vi "RT Main v0.9.vi"() -> ()   [LabVIEW 2017]
doc: "Changelog:\n\nv0.9:\n- Autocycle"
uses:
  Controls/Auto Delays.ctl
  support/Controls/All Inputs.ctl
  support/Controls/Index Details.ctl
  support/Controls/Auto Stats.ctl
  Controls/Auto Times.ctl
  Global Variables/RT GV.vi
  support/Message Queue/Enqueue Message (Single).vi
  Global Variables/FPGA GV.vi
  <vilib>/Utility/error.llb/Error Cluster From Error Code.vi
  <vilib>/rvi/errors/niLvFpgaAdjustHostInterfaceError.vi
  Global Variables/Network Globals.vi
  <vilib>/FPGAPlugInAG/Dynamic/niLvFpga_Close_Dynamic.vi
  <vilib>/rvi/interface/nirviReadWriteControl/nirviReadWriteControl.xnode
  Controls/FPGA Ref.ctl
  <vilib>/rvi/interface/nirviCloseFPGA/nirviCloseFPGA.xnode
  support/Message Queue/Message Queue.lvlib
  NiFpgaLv.dll
  <vilib>/rvi/interface/Simulation/niFpgaSimulationCallBeginRW.vi
panel:
  in  "Auto Para":T1={"Agitator Delays"=[700, 250], "TF Delays"=[700, 800, 2], "Insertion Delays"=[100, 500], "Cutting Delays"=[300, 300, 100], "PF Delays"=[250, 30000], "Measur. Delays"=[500.0, 188.9, 1.0], "Reject Delays"=[500], "BF Delays"=[1000, 1000]}
  in  "Counts in":cluster{"OutputCount":u32, "RejectCount":u32}
  in  "Stop Button 4":bool
  out "error out":errorcluster
  out "Wrong Message":string
  in  "Stop Button":bool
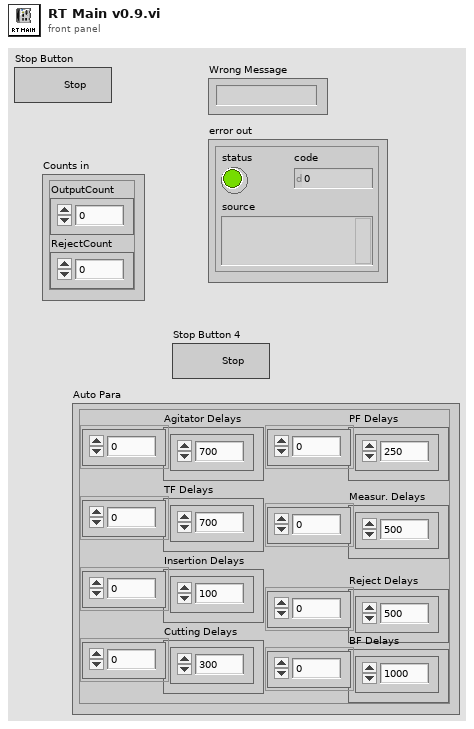
[diagram p1: front panel]
types:
  T1 = typedef "Auto Delays.ctl" = cluster{"Agitator Delays":u32[], "TF Delays":u32[], "Insertion Delays":u32[], "Cutting Delays":u32[], "PF Delays":u32[], "Measur. Delays":dbl[], "Reject Delays":u32[], "BF Delays":u32[]}
  T2 = typedef "FPGA Ref.ctl" = refnum<k20>
  T3 = cluster{"TL_Red":bool, "TL_Orange":bool, "TL_Green":bool, "TL_Buzzer":bool, "SOL_Index_Rotary_CW":bool, "SOL_Index_CNVR_Rotary_CCW":bool, "SOL_Index_CNVR_Stopper_Rear":bool, "SOL_Index_CNVR_Output _Separator _Rear":bool, "Bowl  Feeder_ ON":bool, "Pump_CNVR_Motor _ON":bool, "SOL_Gating_CYL_Rear":bool, "SOL_Tube_Feed_Agitatator":bool, "SOL_Tube_Feed_Gating_CYL":bool, "SOL_Insertion _CYL":bool, "SOL_Insertion_Clamp_CYL":bool, "SOL_Cutting_CYL":bool, "SOL_Cutting_Clamp_CYL":bool, "SOL_Insertion_Air_Nozzle":bool, "SOL_Measurement_CYL":bool, "SOL_Measure_Clamp_CYL":bool, "SOL_Rejection CYL_1":bool, "SOL_Rejection CYL_2":bool, "SOL_Rejection CYL_3":bool, "SOL_Rejection CYL_4":bool, "DO1.24":bool, "DO1.25":bool, "DO1.26":bool, "DO1.27":bool, "DO1.28":bool, "DO1.29":bool, "DO1.30":bool, "DO1.31":bool}
  T4 = typedef "All Inputs.ctl" = cluster{"DI 1":cluster{"Machine_ON":bool, "E_stop ":bool, "SW_Pressure":bool, "SW_Start ":bool, "SW_Reset":bool, "SW_Stop":bool, "SW_Door":bool, "RS_Index_Rotary_CW":bool, "RS_Index_Rotary_CCW":bool, "RS_Index_Stopper _Rear":bool, "RS_Index_Output_Separator_Rear":bool, "PES_Index_Pallet_Sensor":bool, "PES_Index_Output_Part Sensor":bool, "ICS_BF_Low_Level_1":bool, "ICS_BF_Low_Level_2":bool, "ICS_BF_Pump_CNVR_Full_1":bool, "ICS_BF_Pump_CNVR_Full_2":bool, "ICS_BF_Pump_CNVR_Full_3":bool, "ICS_BF_Pump_CNVR_Full_4":bool, "PES_PC_Pump Presence_1":bool, "PES_PC_Pump Presence_2":bool, "PES_PC_Pump Presence_3":bool, "PES_PC_Pump Presence_4":bool, "RS_PC_Gating_Front":bool, "PES_Pump_Interference":bool, "PES_TF_Low_Level":bool, "PES_Tube Presence_1":bool, "PES_Tube Presence_2":bool, "PES_Tube Presence_3":bool, "PES_Tube Presence_4":bool, "DI1.30":bool, "DI1.31":bool}, "DI 2":cluster{"RS_Agitatator_1_Rear ":bool, "RS_Agitatator_2_Rear ":bool, "RS_TF_Gating CYL_Rear":bool, "RS_Insertion_1_Rear":bool, "RS_Insertion_1_Front":bool, "RS_Insertion _2_Rear":bool, "RS_Insertion _2_Front":bool, "RS_Insertion _3_Rear":bool, "RS_Insertion _3_Front":bool, "RS_Insertion _4_Rear":bool, "RS_Insertion _4_Front":bool, "RS_Insertion_Clamp_Rear":bool, "RS_Cutting_Rear":bool, "RS_Cutting_Clamp _Rear":bool, "RS_Measurement_1_Rear":bool, "RS_Measurement_2_Rear":bool, "RS_Measurement_3_Rear":bool, "RS_Measurement_4_Rear":bool, "RS_Measure_Clamp_Rear":bool, "RS_Rejection_1_Rear":bool, "RS_Rejection_2_Rear":bool, "RS_Rejection_3_Rear":bool, "RS_Rejection_4_Rear":bool, "DI2.23":bool, "DI2.24":bool, "DI2.25":bool, "DI2.26":bool, "DI2.27":bool, "DI2.28":bool, "DI2.29":bool, "DI2.30":bool, "DI2.31":bool}, "IAS 1":dbl, "IAS 2":dbl, "IAS 3":dbl, "IAS 4":dbl, "DO 1":cluster{"TL_Red":bool, "TL_Orange":bool, "TL_Green":bool, "TL_Buzzer":bool, "SOL_Index_Rotary_CW":bool, "SOL_Index_CNVR_Rotary_CCW":bool, "SOL_Index_CNVR_Stopper_Rear":bool, "SOL_Index_CNVR_Output _Separator _Rear":bool, "Bowl  Feeder_ ON 1":bool, "Pump_CNVR_Motor _ON":bool, "SOL_PC_Gating_CYL_Rear":bool, "SOL_Tube_Feed_Agitatator":bool, "SOL_Tube_Feed_Gating_CYL":bool, "SOL_Insertion _CYL":bool, "SOL_Insertion_Clamp_CYL":bool, "SOL_Cutting_CYL":bool, "SOL_Cutting_Clamp_CYL":bool, "SOL_Insertion_Air_Nozzle":bool, "SOL_Measurement_CYL":bool, "DO1.19":bool, "SOL_Rejection CYL_1":bool, "SOL_Rejection CYL_2":bool, "SOL_Rejection CYL_3":bool, "SOL_Rejection CYL_4":bool, "Bowl  Feeder_ ON 2":bool, "SOL_BF_BlowerON":bool, "SOL_BF1_Track1":bool, "SOL_BF1_Track2":bool, "SOL_BF2_Track1":bool, "SOL_BF2_Track2":bool, "DO1.30":bool, "DO1.31":bool}}
  T5 = typedef "Index Details.ctl" = cluster{"Time (ms)":u32, "Waveform Graph":i16[]}
  T6 = cluster{T1, "Reject Pallets":cluster{"Reject 1":bool, "Reject 2":bool, "Reject 3":bool, "Reject 4":bool}}
  T7 = typedef "Auto Stats.ctl" = cluster{"Time":timestamp, "OEE":cluster{"AVL":dbl, "PRF":dbl, "QUA":dbl, "OEE":dbl}, "Auto Times":T8, "Counts out":cluster{"OutputCount":u32, "RejectCount":u32}, "Measurements":cluster{"1":dbl, "2":dbl, "3":dbl, "4":dbl}, "Outputs":cluster{"OutputCount":u32, "Numeric Control":u32}}
  T8 = typedef "Auto Times.ctl" = cluster{"Index Time":u32, "TF Time":u32, "Insertion Time":u32, "Cutting Time":u32, "PF Time":u32, "Meas. Time":u32, "Reject Time":u32}
  T9 = cluster{string, dbl, "Counts in":cluster{"OutputCount":u32, "RejectCount":u32}, "Auto Para":T1}
  T10 = cluster{"TL_Red":bool, "TL_Orange":bool, "TL_Green":bool, "TL_Buzzer":bool, "SOL_Index_Rotary_CW":bool, "SOL_Index_CNVR_Rotary_CCW":bool, "SOL_Index_CNVR_Stopper_Rear":bool, "SOL_Index_CNVR_Output _Separator _Rear":bool, "Bowl Feeder_ ON1":bool, "Pump_CNVR_Motor _ON":bool, "SOL_PC_Gating_CYL_Rear":bool, "SOL_Tube_Feed_Agitatator":bool, "SOL_Tube_Feed_Gating_CYL":bool, "SOL_Insertion _CYL":bool, "SOL_Insertion_Clamp_CYL":bool, "SOL_Cutting_CYL":bool, "SOL_Cutting_Clamp_CYL":bool, "SOL_Insertion_Air_Nozzle":bool, "SOL_Measurement_CYL":bool, "DO1.19":bool, "SOL_Rejection CYL_1":bool, "SOL_Rejection CYL_2":bool, "SOL_Rejection CYL_3":bool, "SOL_Rejection CYL_4":bool, "Bowl Feeder_ON2":bool, "SOL_BF_BlowerON":bool, "SOL_BF1_Track1":bool, "SOL_BF1_Track2":bool, "SOL_BF2_Track1":bool, "SOL_BF2_Track2":bool, "DO1.30":bool, "DO1.31":bool}
  T11 = cluster{"Machine_ON":bool, "E_stop ":bool, "SW_Pressure":bool, "SW_Start ":bool, "SW_Reset":bool, "SW_Stop":bool, "SW_Door":bool, "RS_Index_Rotary_CW":bool, "RS_Index_Rotary_CCW":bool, "RS_Index_Stopper _Rear":bool, "RS_Index_Output_Separator_Rear":bool, "PES_Index_Pallet_Sensor":bool, "PES_Index_Output_Part Sensor":bool, "ICS_BF_Low_Level_1":bool, "ICS_BF_Low_Level_2":bool, "ICS_BF_Pump_CNVR_Full_1":bool, "ICS_BF_Pump_CNVR_Full_2":bool, "ICS_BF_Pump_CNVR_Full_3":bool, "ICS_BF_Pump_CNVR_Full_4":bool, "PES_PC_Pump Presence_1":bool, "PES_PC_Pump Presence_2":bool, "PES_PC_Pump Presence_3":bool, "PES_PC_Pump Presence_4":bool, "RS_PC_Gating_Front":bool, "PES_Pump_Interference":bool, "PES_TF_Low_Level":bool, "PES_Tube Presence_1":bool, "PES_Tube Presence_2":bool, "PES_Tube Presence_3":bool, "PES_Tube Presence_4":bool, "DI1.30":bool, "DI1.31":bool}
  T12 = cluster{"RS_Agitatator_1_Rear ":bool, "RS_Agitatator_2_Rear ":bool, "RS_TF_Gating CYL_Rear":bool, "RS_Insertion_1_Rear":bool, "RS_Insertion_1_Front":bool, "RS_Insertion _2_Rear":bool, "RS_Insertion _2_Front":bool, "RS_Insertion _3_Rear":bool, "RS_Insertion _3_Front":bool, "RS_Insertion _4_Rear":bool, "RS_Insertion _4_Front":bool, "RS_Insertion_Clamp_Rear":bool, "RS_Cutting_Rear":bool, "RS_Cutting_Clamp _Rear":bool, "RS_Measurement_1_Rear":bool, "RS_Measurement_2_Rear":bool, "RS_Measurement_3_Rear":bool, "RS_Measurement_4_Rear":bool, "DI2.18":bool, "RS_Rejection_1_Rear":bool, "RS_Rejection_2_Rear":bool, "RS_Rejection_3_Rear":bool, "RS_Rejection_4_Rear":bool, "DI2.23":bool, "DI2.24":bool, "DI2.25":bool, "DI2.26":bool, "DI2.27":bool, "DI2.28":bool, "DI2.29":bool, "DI2.30":bool, "DI2.31":bool}
  T13 = cluster{"Array":string[][], "Machine Status":string}
  T14 = cluster{"Measurements":cluster{"1":dbl, "2":dbl, "3":dbl, "4":dbl}, "Reject Pallets":cluster{"Reject 1":bool, "Reject 2":bool, "Reject 3":bool, "Reject 4":bool}}
  T15 = cluster{"Auto Times":T8, "Results":cluster{"Measurements":cluster{"1":dbl, "2":dbl, "3":dbl, "4":dbl}, "Reject Pallets":cluster{"Reject 1":bool, "Reject 2":bool, "Reject 3":bool, "Reject 4":bool}}, "OutputCount":u32, "error out":errorcluster}
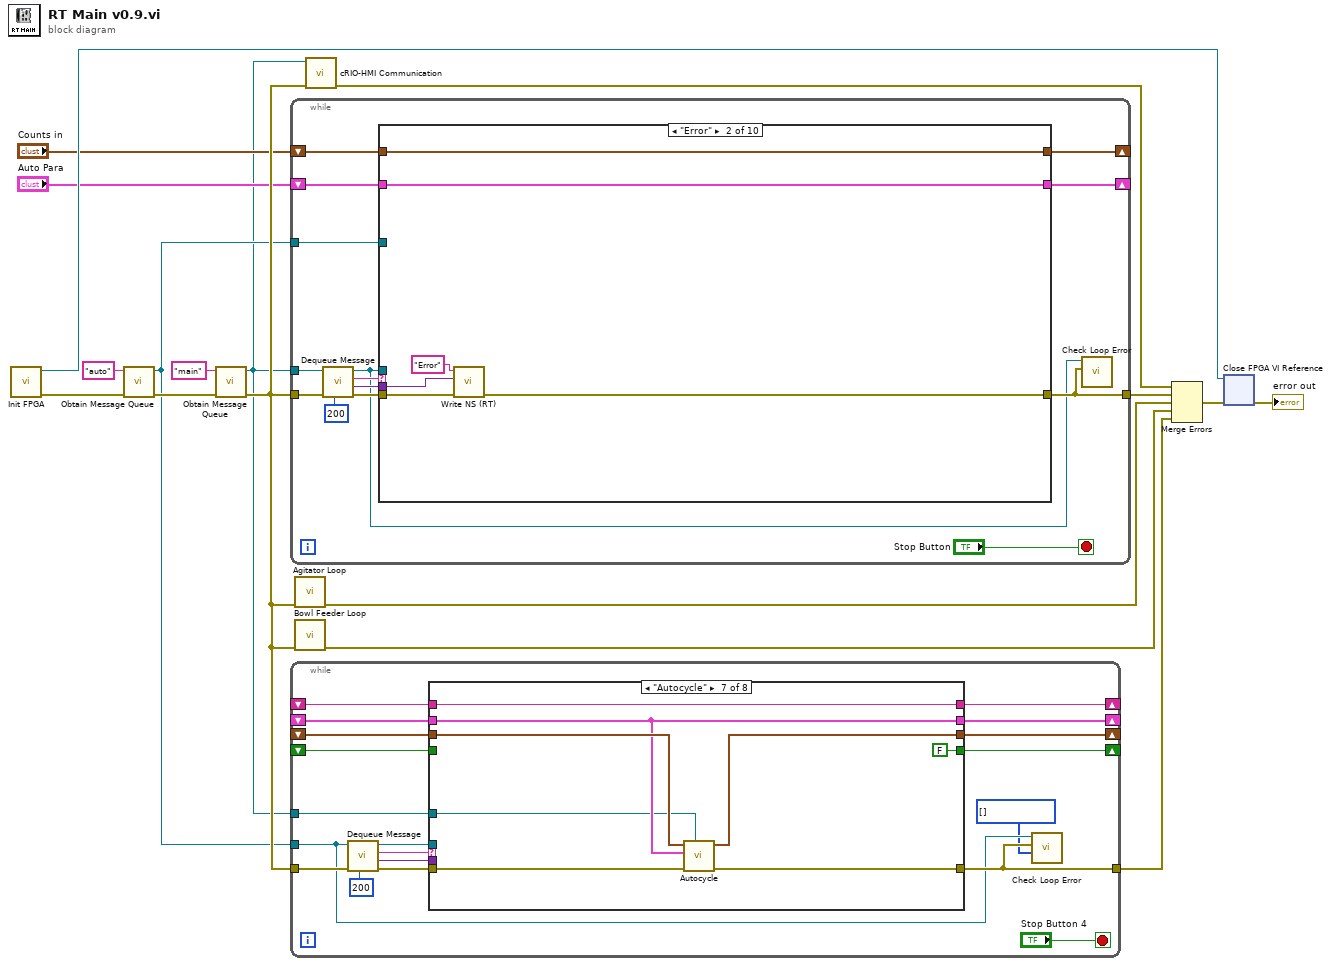
[diagram p0: block diagram]
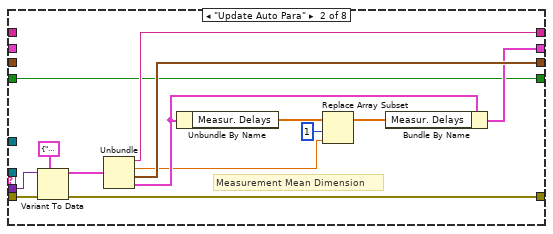
[diagram p3: hidden frame]
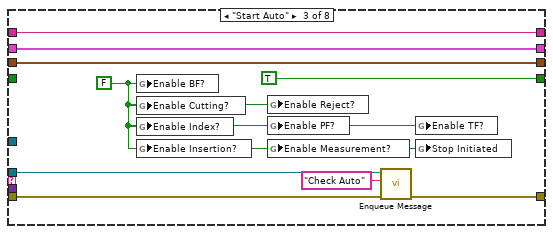
[diagram p4: hidden frame]
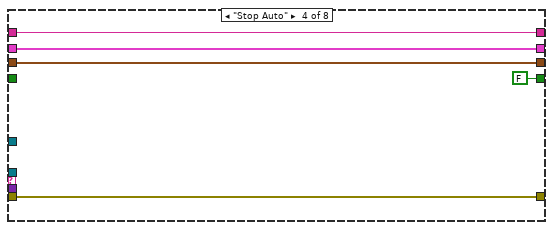
[diagram p5: hidden frame]
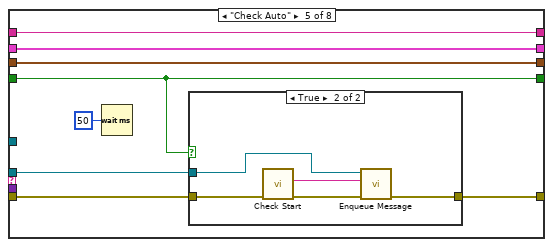
[diagram p6: hidden frame]
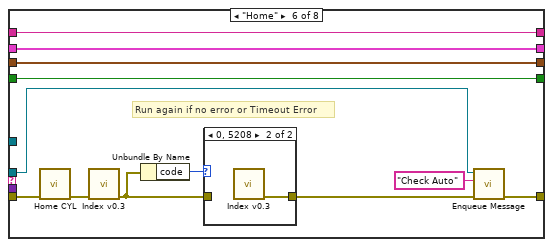
[diagram p8: hidden frame]
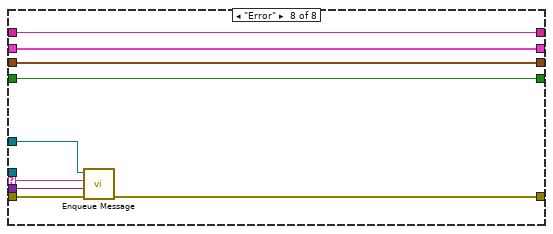
[diagram p10: hidden frame]
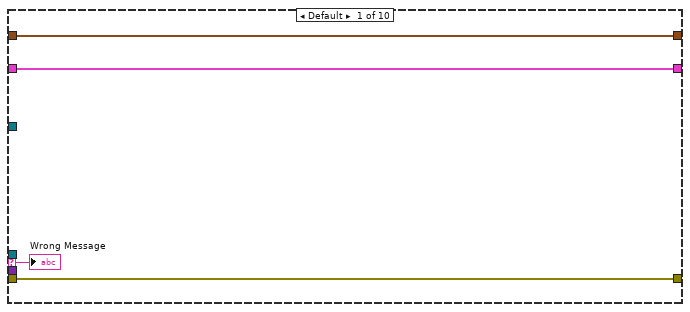
[diagram p11: hidden frame]
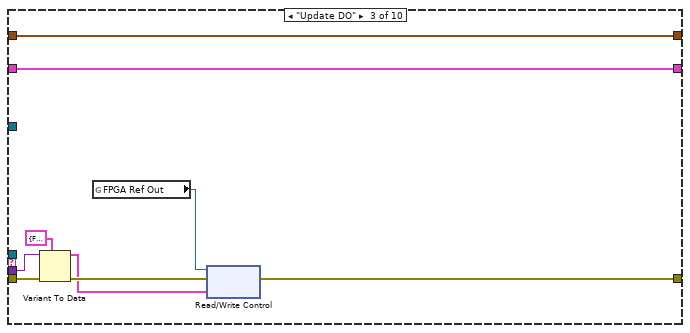
[diagram p12: hidden frame]
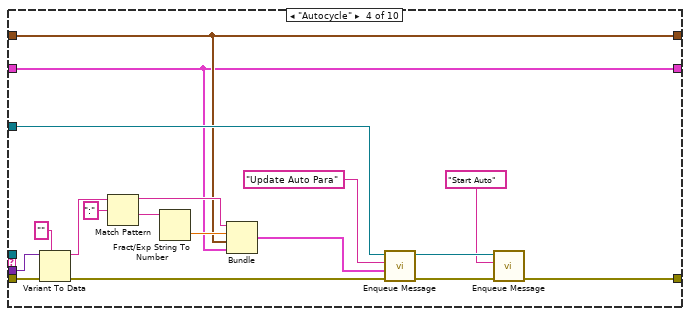
[diagram p13: hidden frame]
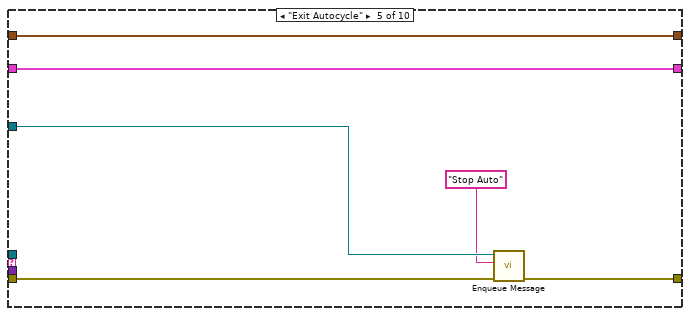
[diagram p14: hidden frame]
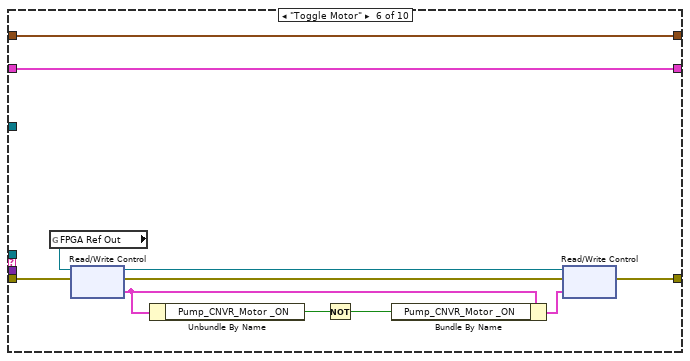
[diagram p15: hidden frame]
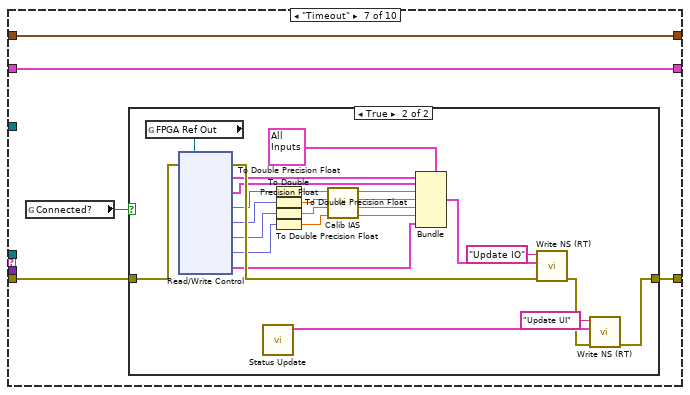
[diagram p16: hidden frame]
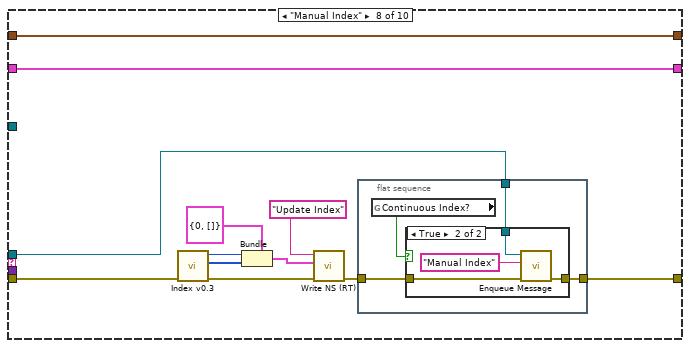
[diagram p18: hidden frame]
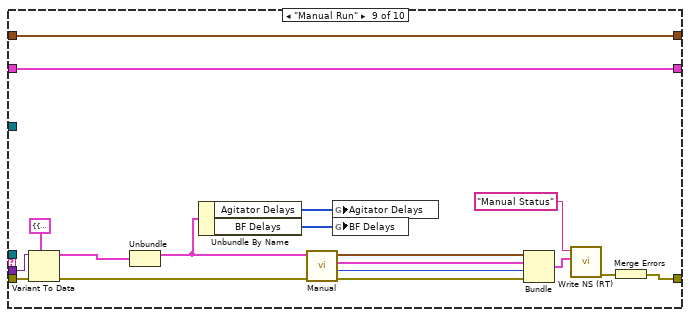
[diagram p20: hidden frame]
diagram:
  n1 = call "Init FPGA.vi"() -> ("error out"=w6:errorcluster, "FPGA Ref Out"=w11:T2)  [unwired: 10 in]
  n2 = call "Obtain Message Queue.vi"("error in (no error)"=w6, "name"="auto") -> ("error out"=w5:errorcluster, "Message Queue"=w2:refnum<queue>)  [unwired: 8 in]
  n3 = call "Obtain Message Queue.vi"("error in (no error)"=w5, "name"="main") -> ("error out"=w10:errorcluster, "Message Queue"=w1:refnum<queue>)  [unwired: 8 in]
  n4 = while {
    tunnel: w10 -> [w30]
    tunnel: w1 -> [w29]
    tunnel: [w25] -> w17
    tunnel: w2 -> [w22]
    shift-right: [w19] -> _
    shift-left: "Auto Para" -> [w20]
    shift-right: [w18] -> _
    shift-left: "Counts in" -> [w21]
    stop <- "Stop Button" stop-if-true
    n5 = call "Dequeue Message.vi"("timeout"=200, "error in (no error)"=w30, "Message Queue"=w29) -> ("error out"=w28:errorcluster, "Message Data"=w26:variant, "Message"=w27:string, "dup Message Queue"=w24:refnum<queue>)  [unwired: 5 in]
    n6 = case shown="\"Error\"" w27 {
      selector: w27 -> [w35 _ _ _ _ _ _ _ _ _]
      tunnel: w28 -> [w34 w39 w50 w68 w74 w84 w89 w128 w155 w165]
      tunnel: w24 -> [_ _ _ _ _ _ _ w120 _ _]
      tunnel: w26 -> [_ w37 w49 w67 _ _ _ _ w154 w164]
      tunnel: [w34 w38 w45 w53 w70 w82 w90 w121 w150 w161] -> w25
      tunnel: w22 -> [_ _ _ w60 w73 _ _ _ _ _]
      tunnel: w21 -> [w33 w41 w43 w57 w72 w76 w87 w117 w141 w160]
      tunnel: w20 -> [w32 w40 w42 w56 w71 w75 w86 w118 w140 w159]
      tunnel: [w32 w40 w42 w56 w71 w75 w86 w118 w140 w159] -> w19
      tunnel: [w33 w41 w43 w57 w72 w76 w87 w117 w141 w160] -> w18
      frame Default {
        "Wrong Message" <- w35
      }
      frame "Error" {
        n7 = call "Write NS (RT).vi"("error in (no error)"=w39, "Message Data"=w37, "Message"="Error") -> ("error out"=w38:errorcluster)  [unwired: 8 in]
      }
      frame "Update DO" {
        n8 = Variant To Data(error in=w50, type=T3 {"TL_Red"=FALSE, "TL_Orange"=FALSE, "TL_Green"=FALSE, "TL_Buzzer"=FALSE, "SOL_Index_Rotary_CW"=FALSE, "SOL_Index_CNVR_Rotary_CCW"=FALSE, "SOL_Index_CNVR_Stopper_Rear"=FALSE, "SOL_Index_CNVR_Output _Separator _Rear"=FALSE, "Bowl  Feeder_ ON"=FALSE, "Pump_CNVR_Motor _ON"=FALSE, "SOL_Gating_CYL_Rear"=FALSE, "SOL_Tube_Feed_Agitatator"=FALSE, "SOL_Tube_Feed_Gating_CYL"=FALSE, "SOL_Insertion _CYL"=FALSE, "SOL_Insertion_Clamp_CYL"=FALSE, "SOL_Cutting_CYL"=FALSE, "SOL_Cutting_Clamp_CYL"=FALSE, "SOL_Insertion_Air_Nozzle"=FALSE, "SOL_Measurement_CYL"=FALSE, "SOL_Measure_Clamp_CYL"=FALSE, "SOL_Rejection CYL_1"=FALSE, "SOL_Rejection CYL_2"=FALSE, "SOL_Rejection CYL_3"=FALSE, "SOL_Rejection CYL_4"=FALSE, "DO1.24"=FALSE, "DO1.25"=FALSE, "DO1.26"=FALSE, "DO1.27"=FALSE, "DO1.28"=FALSE, "DO1.29"=FALSE, "DO1.30"=FALSE, "DO1.31"=FALSE} ("DO 1"), Variant=w49) -> (data=w44:T3, error out=w46:errorcluster)
        n9 = global read "FPGA GV.vi" "FPGA Ref Out"() -> (w47:T2)
        n10 = xnode "Read/Write Control"("FPGA VI Reference In"=w47, "error in"=w46, "DO 1"=w44) -> ("error out"=w45:errorcluster)  [unwired: 1 out]
      }
      frame "Autocycle" {
        n11 = Variant To Data(error in=w68, type="", Variant=w67) -> (data=w63:string, error out=w61:errorcluster)
        n12 = Match Pattern(string=w63, regular expression=":") -> (before substring=w59:string, after substring=w64:string)  [unwired: 1 in, 2 out]
        n13 = Fract/Exp String To Number(string=w64) -> (number=w58:dbl)  [unwired: 3 in, 1 out]
        n14 = Bundle(w59, w58, "Counts in"=w57, "Auto Para"=w56) -> (w55:T9)  [unwired: 1 in]
        n15 = call-poly "Enqueue Message.vi"("error in (no error)"=w61, "Message Data"=w55, "Message"="Update Auto Para", "Message Queue"=w60) -> ("error out"=w54:errorcluster, "dup Message Queue"=w52:refnum<queue>)  [unwired: 6 in]
        n16 = call-poly "Enqueue Message.vi"("error in (no error)"=w54, "Message"="Start Auto", "Message Queue"=w52) -> ("error out"=w53:errorcluster)  [unwired: 7 in, 1 out]
      }
      frame "Exit Autocycle" {
        n17 = call-poly "Enqueue Message.vi"("error in (no error)"=w74, "Message"="Stop Auto", "Message Queue"=w73) -> ("error out"=w70:errorcluster)  [unwired: 7 in, 1 out]
      }
      frame "Toggle Motor" {
        n18 = global read "FPGA GV.vi" "FPGA Ref Out"() -> (w85:T2)
        n19 = xnode "Read/Write Control"("FPGA VI Reference In"=w85, "error in"=w84) -> ("FPGA VI Reference Out"=w81:T2, "error out"=w83:errorcluster, "DO 1"=w79:T10)
        n20 = Unbundle By Name(w79) -> ("Pump_CNVR_Motor _ON"=w80:bool)
        n21 = Not(x=w80) -> (.not. x?=w77:bool)
        n22 = Bundle By Name(cluster=w79, "Pump_CNVR_Motor _ON"=w77) -> (w78:T10)
        n23 = xnode "Read/Write Control"("FPGA VI Reference In"=w81, "error in"=w83, "DO 1"=w78) -> ("error out"=w82:errorcluster)  [unwired: 1 out]
      }
      frame "Timeout" {
        n24 = global read "Network Globals.vi" "Connected?"() -> (w88:bool)
        n25 = case shown="True" w88 {
          tunnel: [w91 w93] -> w90
          tunnel: w89 -> [w91 w115]
          frame False {
          }
          frame True {
            n26 = global read "FPGA GV.vi" "FPGA Ref Out"() -> (w92:T2)
            n27 = xnode "Read/Write Control"("FPGA VI Reference In"=w92, "error in"=w115) -> ("error out"=w114:errorcluster, "DI 1"=w113:T11, "DI 2"=w112:T12, "AI0"=w111:fxp<+/-,27,6>, "AI1"=w110:fxp<+/-,27,6>, "AI2"=w109:fxp<+/-,27,6>, "AI3"=w108:fxp<+/-,27,6>, "DO 1"=w105:T10)  [unwired: 1 out]
            n28 = call "Status Update.vi"() -> ("Status Cluster"=w95:T13)  [unwired: 11 in]
            n29 = To Double Precision Float(number=w111) -> (double precision float=w98:dbl)
            n30 = To Double Precision Float(number=w110) -> (double precision float=w100:dbl)
            n31 = To Double Precision Float(number=w109) -> (double precision float=w102:dbl)
            n32 = To Double Precision Float(number=w108) -> (double precision float=w104:dbl)
            n33 = call "Calib IAS.vi"("x 4"=w104, "x 3"=w102, "x 2"=w100, "x"=w98) -> ("y 4"=w103:dbl, "y 3"=w101:dbl, "y 2"=w99:dbl, "y 1"=w97:dbl)  [unwired: 4 in]
            n34 = Bundle(cluster=T4 {"DI 1"={"Machine_ON"=FALSE, "E_stop "=FALSE, "SW_Pressure"=FALSE, "SW_Start "=FALSE, "SW_Reset"=FALSE, "SW_Stop"=FALSE, "SW_Door"=FALSE, "RS_Index_Rotary_CW"=FALSE, "RS_Index_Rotary_CCW"=FALSE, "RS_Index_Stopper _Rear"=FALSE, "RS_Index_Output_Separator_Rear"=FALSE, "PES_Index_Pallet_Sensor"=FALSE, "PES_Index_Output_Part Sensor"=FALSE, "ICS_BF_Low_Level_1"=FALSE, "ICS_BF_Low_Level_2"=FALSE, "ICS_BF_Pump_CNVR_Full_1"=FALSE, "ICS_BF_Pump_CNVR_Full_2"=FALSE, "ICS_BF_Pump_CNVR_Full_3"=FALSE, "ICS_BF_Pump_CNVR_Full_4"=FALSE, "PES_PC_Pump Presence_1"=FALSE, "PES_PC_Pump Presence_2"=FALSE, "PES_PC_Pump Presence_3"=FALSE, "PES_PC_Pump Presence_4"=FALSE, "RS_PC_Gating_Front"=FALSE, "PES_Pump_Interference"=FALSE, "PES_TF_Low_Level"=FALSE, "PES_Tube Presence_1"=FALSE, "PES_Tube Presence_2"=FALSE, "PES_Tube Presence_3"=FALSE, "PES_Tube Presence_4"=FALSE, "DI1.30"=FALSE, "DI1.31"=FALSE}, "DI 2"={"RS_Agitatator_1_Rear "=FALSE, "RS_Agitatator_2_Rear "=FALSE, "RS_TF_Gating CYL_Rear"=FALSE, "RS_Insertion_1_Rear"=FALSE, "RS_Insertion_1_Front"=FALSE, "RS_Insertion _2_Rear"=FALSE, "RS_Insertion _2_Front"=FALSE, "RS_Insertion _3_Rear"=FALSE, "RS_Insertion _3_Front"=FALSE, "RS_Insertion _4_Rear"=FALSE, "RS_Insertion _4_Front"=FALSE, "RS_Insertion_Clamp_Rear"=FALSE, "RS_Cutting_Rear"=FALSE, "RS_Cutting_Clamp _Rear"=FALSE, "RS_Measurement_1_Rear"=FALSE, "RS_Measurement_2_Rear"=FALSE, "RS_Measurement_3_Rear"=FALSE, "RS_Measurement_4_Rear"=FALSE, "RS_Measure_Clamp_Rear"=FALSE, "RS_Rejection_1_Rear"=FALSE, "RS_Rejection_2_Rear"=FALSE, "RS_Rejection_3_Rear"=FALSE, "RS_Rejection_4_Rear"=FALSE, "DI2.23"=FALSE, "DI2.24"=FALSE, "DI2.25"=FALSE, "DI2.26"=FALSE, "DI2.27"=FALSE, "DI2.28"=FALSE, "DI2.29"=FALSE, "DI2.30"=FALSE, "DI2.31"=FALSE}, "IAS 1"=0.0, "IAS 2"=0.0, "IAS 3"=0.0, "IAS 4"=0.0, "DO 1"={"TL_Red"=FALSE, "TL_Orange"=FALSE, "TL_Green"=FALSE, "TL_Buzzer"=FALSE, "SOL_Index_Rotary_CW"=FALSE, "SOL_Index_CNVR_Rotary_CCW"=FALSE, "SOL_Index_CNVR_Stopper_Rear"=FALSE, "SOL_Index_CNVR_Output _Separator _Rear"=FALSE, "Bowl  Feeder_ ON 1"=FALSE, "Pump_CNVR_Motor _ON"=FALSE, "SOL_PC_Gating_CYL_Rear"=FALSE, "SOL_Tube_Feed_Agitatator"=FALSE, "SOL_Tube_Feed_Gating_CYL"=FALSE, "SOL_Insertion _CYL"=FALSE, "SOL_Insertion_Clamp_CYL"=FALSE, "SOL_Cutting_CYL"=FALSE, "SOL_Cutting_Clamp_CYL"=FALSE, "SOL_Insertion_Air_Nozzle"=FALSE, "SOL_Measurement_CYL"=FALSE, "DO1.19"=FALSE, "SOL_Rejection CYL_1"=FALSE, "SOL_Rejection CYL_2"=FALSE, "SOL_Rejection CYL_3"=FALSE, "SOL_Rejection CYL_4"=FALSE, "Bowl  Feeder_ ON 2"=FALSE, "SOL_BF_BlowerON"=FALSE, "SOL_BF1_Track1"=FALSE, "SOL_BF1_Track2"=FALSE, "SOL_BF2_Track1"=FALSE, "SOL_BF2_Track2"=FALSE, "DO1.30"=FALSE, "DO1.31"=FALSE}}, "DI 1"=w113, "DI 2"=w112, "IAS 1"=w97, "IAS 2"=w99, "IAS 3"=w101, "IAS 4"=w103, "DO 1"=w105) -> (w107:T4)
            n35 = call "Write NS (RT).vi"("error in (no error)"=w114, "Message Data"=w107, "Message"="Update IO") -> ("error out"=w94:errorcluster)  [unwired: 8 in]
            n36 = call "Write NS (RT).vi"("error in (no error)"=w94, "Message Data"=w95, "Message"="Update UI") -> ("error out"=w93:errorcluster)  [unwired: 8 in]
          }
        }
      }
      frame "Manual Index" {
        n37 = call "Index v0.3.vi"("error in (no error)"=w128) -> ("error out"=w126:errorcluster, "Waveform Graph"=w124:i16[], "Index Time"=w125:u32)  [unwired: 7 in, 1 out]
        n38 = Bundle(cluster=T5 {"Time (ms)"=0, "Waveform Graph"=[]}, "Time (ms)"=w125, "Waveform Graph"=w124) -> (w123:T5)
        n39 = call "Write NS (RT).vi"("error in (no error)"=w126, "Message Data"=w123, "Message"="Update Index") -> ("error out"=w122:errorcluster)  [unwired: 8 in]
        n40 = flat-sequence {
          tunnel: w122 -> [w132]
          tunnel: [w131] -> w121
          tunnel: w120 -> [w129]
          frame #0 {
            n41 = global read "RT GV.vi" "Continuous Index?"() -> (w130:bool)
            n42 = case shown="True" w130 {
              tunnel: w132 -> [w133 w137]
              tunnel: [w133 w136] -> w131
              tunnel: w129 -> [_ w134]
              frame False {
              }
              frame True {
                n43 = call-poly "Enqueue Message.vi"("error in (no error)"=w137, "Message"="Manual Index", "Message Queue"=w134) -> ("error out"=w136:errorcluster)  [unwired: 7 in, 1 out]
              }
            }
          }
        }
      }
      frame "Manual Run" {
        n44 = Variant To Data(error in=w155, type=T6 {{"Agitator Delays"=[1000], "TF Delays"=[1000], "Insertion Delays"=[1000], "Cutting Delays"=[1000], "PF Delays"=[1000], "Measur. Delays"=[1000.0], "Reject Delays"=[1000], "BF Delays"=[1000]}, "Reject Pallets"={"Reject 1"=FALSE, "Reject 2"=FALSE, "Reject 3"=FALSE, "Reject 4"=FALSE}}, Variant=w154) -> (data=w146:T6, error out=w153:errorcluster)
        n45 = Unbundle(w146) -> (w143:T1)  [unwired: 1 out]
        n46 = Unbundle By Name(w143) -> ("Agitator Delays"=w139:u32[], "BF Delays"=w138:u32[])
        n47 = call "Manual.vi"("error in"=w153, "Auto Delays"=w143) -> ("error out"=w145:errorcluster, "OutputCount"=w144:u32, "Results"=w142:T14, "Auto Times"=w149:T8)  [unwired: 6 in]
        n48 = global write "RT GV.vi" "Agitator Delays"(w139) -> ()
        n49 = global write "RT GV.vi" "BF Delays"(w138) -> ()
        n50 = Bundle("Auto Times"=w149, "Results"=w142, "OutputCount"=w144, "error out"=w145) -> (w148:T15)  [unwired: 1 in]
        n51 = call "Write NS (RT).vi"("Message Data"=w148, "Message"="Manual Status") -> ("error out"=w151:errorcluster)  [unwired: 9 in]
        n52 = Merge Errors(w151) -> (w150:errorcluster)
      }
      frame "Log Cycle" {
        n53 = Variant To Data(error in=w165, type=T7 {"Time"=timestamp(0 s since 1904-01-01), "OEE"={"AVL"=100.0, "PRF"=100.0, "QUA"=100.0, "OEE"=0.0}, "Auto Times"={"Index Time"=0, "TF Time"=0, "Insertion Time"=0, "Cutting Time"=0, "PF Time"=0, "Meas. Time"=0, "Reject Time"=0}, "Counts out"={"OutputCount"=0, "RejectCount"=0}, "Measurements"={"1"=0.0, "2"=0.0, "3"=0.0, "4"=0.0}, "Outputs"={"OutputCount"=0, "Numeric Control"=0}} ("Auto Stats"), Variant=w164) -> (data=w156:T7, error out=w157:errorcluster)
        n54 = call "Write NS (RT).vi"("error in (no error)"=w157, "Message Data"=w156, "Message"="Autocycle Log") -> ("error out"=w162:errorcluster)  [unwired: 8 in]
        n55 = Merge Errors(w162) -> (w161:errorcluster)
      }
    }
    n56 = call "Check Loop Error.vi"("error to process"=w25, "Message Queue"=w24) -> ()  [unwired: 8 in, 2 out]
  }
  n57 = while {
    tunnel: w10 -> [w180]
    tunnel: [w178] -> w9
    shift-right: [w182] -> _
    shift-left: _ -> [w183]
    tunnel: w2 -> [w170]
    shift-right: [w174] -> _
    shift-left: _ -> [w173]
    shift-right: [w172] -> _
    shift-left: _ -> [w171]
    shift-right: [w169] -> _
    shift-left: _ -> [w168]
    tunnel: w1 -> [w167]
    stop <- "Stop Button 4" stop-if-true
    n58 = call "Dequeue Message.vi"("timeout"=200, "error in (no error)"=w180, "Message Queue"=w170) -> ("error out"=w179:errorcluster, "Message Data"=w175:variant, "Message"=w176:string, "dup Message Queue"=w177:refnum<queue>)  [unwired: 5 in]
    n59 = case shown="\"Autocycle\"" w176 {
      selector: w176 -> [_ _ _ _ _ _ _ w258]
      tunnel: w179 -> [w189 w203 w208 w214 w220 w239 w253 w256]
      tunnel: [w189 w202 w207 w214 w222 w234 w252 w255] -> w178
      tunnel: w183 -> [w188 _ w212 w217 w225 w243 w251 w262]
      tunnel: [w188 w197 w212 w217 w225 w243 w250 w262] -> w182
      tunnel: w177 -> [_ _ w206 _ w221 w232 _ _]
      tunnel: w175 -> [_ w201 _ _ _ _ _ w257]
      tunnel: [w187 w198 w211 w216 w224 w242 w249 w261] -> w174
      tunnel: w173 -> [w187 _ w211 w216 w224 w242 w249 w261]
      tunnel: [w186 w191 w210 w215 w223 w241 w247 w260] -> w172
      tunnel: w171 -> [w186 _ w210 w215 w223 w241 w247 w260]
      tunnel: [w185 w190 TRUE FALSE w219 w240 FALSE w259] -> w169
      tunnel: w168 -> [w185 w190 _ _ w219 w240 _ w259]
      tunnel: w167 -> [_ _ _ _ _ _ w246 w254]
      frame Default {
      }
      frame "Update Auto Para" {
        # "Measurement Mean Dimension"
        n60 = Variant To Data(error in=w203, type=T9 {"", 0.0, "Counts in"={"OutputCount"=0, "RejectCount"=0}, "Auto Para"={"Agitator Delays"=[], "TF Delays"=[], "Insertion Delays"=[], "Cutting Delays"=[], "PF Delays"=[], "Measur. Delays"=[], "Reject Delays"=[], "BF Delays"=[]}} ("cluster"), Variant=w201) -> (data=w199:T9, error out=w202:errorcluster)
        n61 = Unbundle(w199) -> (w198:string, w193:dbl, "Counts in"=w197:cluster{"OutputCount":u32, "RejectCount":u32}, "Auto Para"=w196:T1)
        n62 = Unbundle By Name(w196) -> ("Measur. Delays"=w195:dbl[])
        n63 = Replace Array Subset(array=w195, new element=w193, index=1) -> (w192:dbl[])
        n64 = Bundle By Name(cluster=w196, "Measur. Delays"=w192) -> (w191:T1)
      }
      frame "Start Auto" {
        w204 = FALSE ("Enable BF?")
        n65 = global write "RT GV.vi" "Enable BF?"(w204) -> ()
        n66 = global write "RT GV.vi" "Enable Cutting?"(w204) -> ()
        n67 = global write "RT GV.vi" "Enable Index?"(w204) -> ()
        n68 = global write "RT GV.vi" "Enable Insertion?"(w204) -> ()
        n69 = global write "RT GV.vi" "Enable Reject?"(w204) -> ()
        n70 = global write "RT GV.vi" "Enable PF?"(w204) -> ()
        n71 = global write "RT GV.vi" "Enable Measurement?"(w204) -> ()
        n72 = call-poly "Enqueue Message.vi"("error in (no error)"=w208, "Message"="Check Auto", "Message Queue"=w206) -> ("error out"=w207:errorcluster)  [unwired: 7 in, 1 out]
        n73 = global write "RT GV.vi" "Enable TF?"(w204) -> ()
        n74 = global write "RT GV.vi" "Stop Initiated"(w204) -> ()
      }
      frame "Stop Auto" {
      }
      frame "Check Auto" {
        n75 = Wait (ms)(milliseconds to wait=u32 50) -> ()  [unwired: 1 out]
        n76 = case shown="True" w219 {
          tunnel: [w226 w231] -> w222
          tunnel: w221 -> [_ w227]
          tunnel: w220 -> [w226 w230]
          frame False {
          }
          frame True {
            n77 = call "Check Start.vi"("error in"=w230) -> ("error out"=w229:errorcluster, "Message"=w228:string)  [unwired: 9 in]
            n78 = call-poly "Enqueue Message.vi"("error in (no error)"=w229, "Message"=w228, "Message Queue"=w227) -> ("error out"=w231:errorcluster)  [unwired: 7 in, 1 out]
          }
        }
      }
      frame "Home" {
        # "Run again if no error or Timeout Error"
        n79 = call "Home CYL.vi"("error in"=w239) -> ("error out"=w238:errorcluster)  [unwired: 10 in]
        n80 = call "Index v0.3.vi"("error in (no error)"=w238) -> ("error out"=w236:errorcluster)  [unwired: 7 in, 3 out]
        n81 = Unbundle By Name(w236) -> ("code"=w237:i32)
        n82 = case shown="0, 5208" w237 {
          tunnel: [w244 w245] -> w233
          tunnel: w236 -> [w244 _]
          frame Default {
          }
          frame 0, 5208 {
            n83 = call "Index v0.3.vi"() -> ("error out"=w245:errorcluster)  [unwired: 8 in, 3 out]
          }
        }
        n84 = call-poly "Enqueue Message.vi"("error in (no error)"=w233, "Message"="Check Auto", "Message Queue"=w232) -> ("error out"=w234:errorcluster)  [unwired: 7 in, 1 out]
      }
      frame "Autocycle" {
        n85 = call "Autocycle.vi"("Message Queue"=w246, "error in"=w253, "Auto Para"=w247, "Counts in"=w251) -> ("error out"=w252:errorcluster, "Counts out"=w250:cluster{"OutputCount":u32, "RejectCount":u32})  [unwired: 6 in]
      }
      frame "Error" {
        n86 = call-poly "Enqueue Message.vi"("error in (no error)"=w256, "Message Data"=w257, "Message"=w258, "Message Queue"=w254) -> ("error out"=w255:errorcluster)  [unwired: 6 in, 1 out]
      }
    }
    n87 = call "Check Loop Error.vi"("Ignore Errors"=i32[] [], "error to process"=w178, "Message Queue"=w170) -> ()  [unwired: 7 in, 2 out]
  }
  n88 = call "Agitator Loop.vi"("error in (no error)"=w10) -> ("error out"=w13:errorcluster)  [unwired: 10 in]
  n89 = call "Bowl Feeder Loop.vi"("error in (no error)"=w10) -> ("error out"=w12:errorcluster)  [unwired: 10 in]
  n90 = call "cRIO-HMI Communication.vi"("error in (no error)"=w10, "Message Queue"=w1) -> ("error out"=w16:errorcluster)  [unwired: 9 in]
  n91 = Merge Errors(w16, w17, w13, w12, w9) -> (w15:errorcluster)
  n92 = xnode ("Close FPGA VI Reference")("FPGA VI Reference In"=w11, "error in"=w15) -> ("error out"=→"error out":errorcluster)
